vi "arrayCEXT.vi"(2 "Array In":cxt[](array[numeric]) format="%.2f", 3 "Base":cxt format="%.2f") -> (0 "Array Out (not in place)":cxt[](array[numeric]) format="%.2f", 1 "Array Out":cxt[](array[numeric]) format="%.2f")   [LabVIEW 2013]
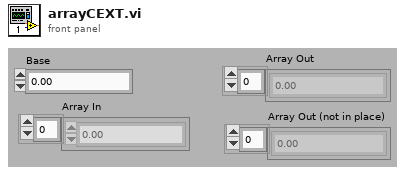
[diagram p1: front panel]
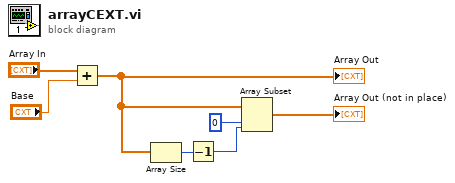
[diagram p0: block diagram]
diagram:
  n1 = Add(x="Array In", y="Base") -> (x+y=w1:cxt[])
  "Array Out" <- w1
  n2 = Array Size(array=w1) -> (size(s)=w5:i32)
  n3 = Decrement(x=w5) -> (x-1=w6:i32)
  n4 = Array Subset(array=w1, index=0, length=w6) -> (→"Array Out (not in place)":cxt[])
